vi "Remove Connection from State.vi"(8 "error in (no error)":errorcluster, 9 "Connection":T1, 10 "State":string, 11 "Channel Ref in":T2 format="%.0x") -> (0 "error out":errorcluster, 1 "connection found":bool, 3 "Channel Ref out":T2=18446744073709551615 format="%.0x")   [LabVIEW 2017, in "SLSC Switch Scripting.lvlib"]
uses:
  SLSC Switch Scripting.lvlib
  <vilib>/NI Veristand/Custom Device API/Custom Device Item Ref.ctl
  Connection.ctl
  NationalInstruments.VeriStand.SystemDefinitionAPI
  SLSC Scripting Constants.vi
  <vilib>/NI VeriStand/Custom Device API/Custom Device API.lvlib
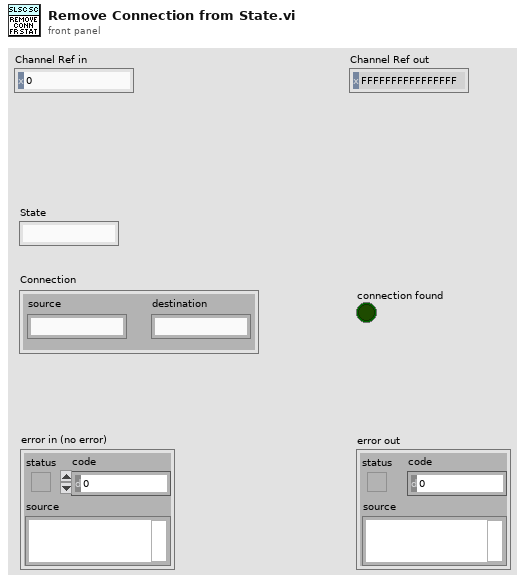
[diagram p1: front panel]
types:
  T1 = typedef "SLSC Switch Scripting.lvlib/Connection.ctl" = cluster{"source":string, "destination":string}
  T2 = typedef "Custom Device API.lvlib/Custom Device Item Ref.ctl" = u64
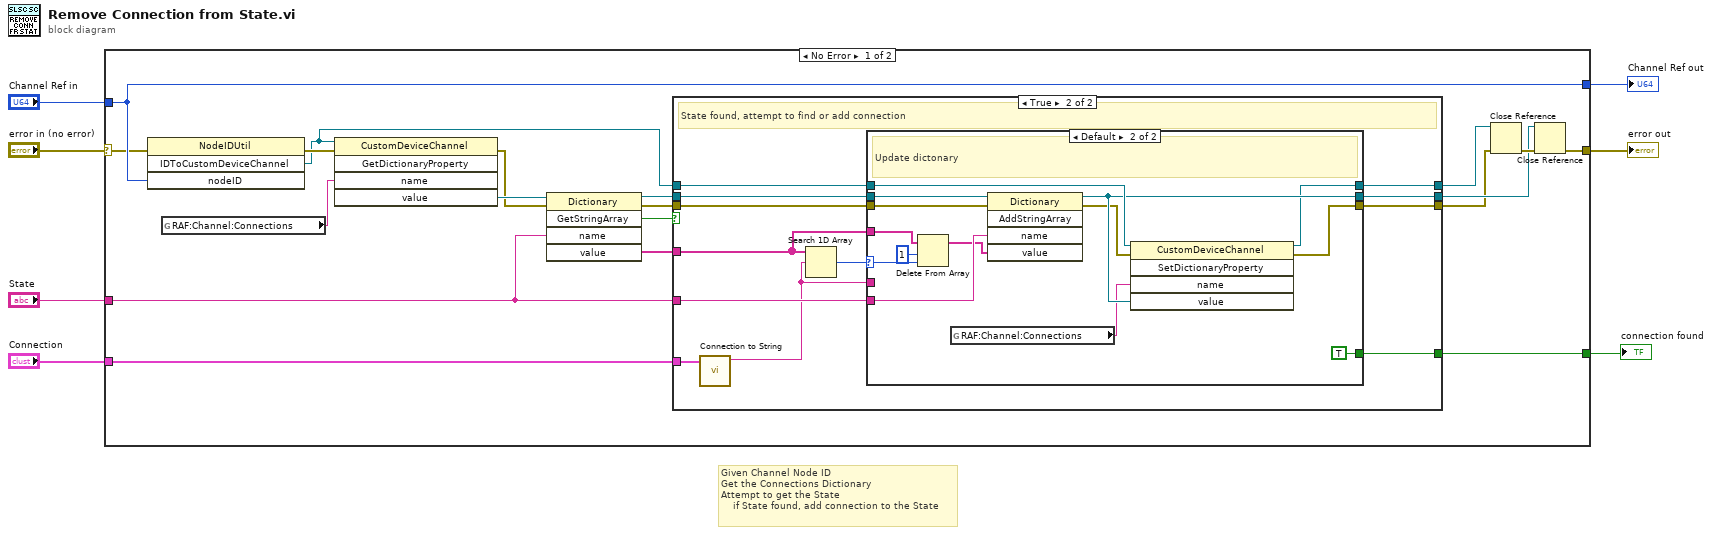
[diagram p0: block diagram]
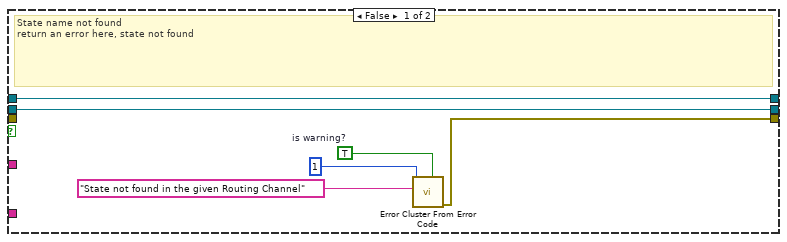
[diagram p2: hidden frame]
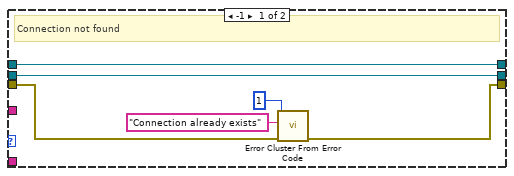
[diagram p3: hidden frame]
diagram:
  # "Given Channel Node ID\nGet the Connections Dictionary\nAttempt to get the State\n    if State found, add connection to the State"
  n1 = case shown="No Error" "error in (no error)" {
    selector: "error in (no error)" -> [w22 w66]
    tunnel: [w26 w66] -> w6
    tunnel: "Channel Ref in" -> [w23 w65]
    tunnel: [w23 w65] -> w4
    tunnel: "State" -> [w15 _]
    tunnel: [w10 _] -> w2
    tunnel: "Connection" -> [w9 _]
    frame No Error {
      n2 = invoke class="NodeIDUtil" method="IDToCustomDeviceChannel"(error in=w22, "nodeID"=w23) -> (error out=w24:errorcluster, "IDToCustomDeviceChannel"=w12:refnum<k24>)  [unwired: 2 in, 2 out]
      n3 = global read "SLSC Scripting Constants.vi" "RAF:Channel:Connections"() -> (w8:string)
      n4 = invoke class="CustomDeviceChannel" method="GetDictionaryProperty"(reference=w12, error in=w24, "name"=w8) -> (error out=w19:errorcluster, "value"=w20:refnum<k24>)  [unwired: 2 in, 3 out]
      n5 = invoke class="Dictionary" method="GetStringArray"(reference=w20, error in=w19, "name"=w15) -> (reference out=w16:refnum<k24>, error out=w17:errorcluster, "GetStringArray"=w18:bool, "value"=w21:string[])  [unwired: 2 in, 1 out]
      n6 = case shown="True" w18 {
        tunnel: w21 -> [_ w36]
        tunnel: w17 -> [_ w43]
        tunnel: [w29 w42] -> w13
        tunnel: w15 -> [_ w41]
        tunnel: w16 -> [w28 w40]
        tunnel: [w28 w39] -> w14
        tunnel: w12 -> [w27 w38]
        tunnel: [w27 w37] -> w11
        tunnel: [_ w35] -> w10
        tunnel: w9 -> [_ w34]
        frame False {
          w31 = TRUE  # is warning?
          # "State name not found\nreturn an error here, state not found"
          n7 = call <vilib>:"Error Cluster From Error Code.vi"("is warning? (False)"=w31, "error message (\"\")"="State not found in the given Routing Channel" ("error message (\"\")"), "error code (0)"=1) -> ("error out"=w29:errorcluster)  [unwired: 6 in]
        }
        frame True {
          # "State found, attempt to find or add connection"
          n8 = call "Connection to String.vi"("Connection"=w34) -> ("String"=w33:string)  [unwired: 10 in]
          n9 = Search 1D Array(1D array=w36, element=w33) -> (index of element=w44:i32)  [unwired: 1 in]
          n10 = case shown="Default" w44 {
            selector: w44 -> [_ w56]
            tunnel: w43 -> [w48 w55]
            tunnel: [w47 w59] -> w42
            tunnel: w41 -> [_ w64]
            tunnel: w40 -> [w46 w63]
            tunnel: [w46 w61] -> w39
            tunnel: w38 -> [w45 w62]
            tunnel: [w45 w58] -> w37
            tunnel: w36 -> [_ w57]
            tunnel: w33 -> [_ _]
            tunnel: [_ TRUE] -> w35
            frame -1 {
              # "Connection not found"
              n11 = call <vilib>:"Error Cluster From Error Code.vi"("error in (no error)"=w48, "error message (\"\")"="Connection already exists" ("error message (\"\")"), "error code (0)"=1) -> ("error out"=w47:errorcluster)  [unwired: 6 in]
            }
            frame Default {
              # "Update dictonary"
              n12 = Delete From Array(array=w57, length=1, index=w56) -> (array with subset deleted=w54:string[])  [unwired: 1 out]
              n13 = global read "SLSC Scripting Constants.vi" "RAF:Channel:Connections"() -> (w51:string)
              n14 = invoke class="Dictionary" method="AddStringArray"(reference=w63, error in=w55, "name"=w64, "value"=w54) -> (reference out=w61:refnum<k24>, error out=w60:errorcluster)  [unwired: 1 in, 3 out]
              n15 = invoke class="CustomDeviceChannel" method="SetDictionaryProperty"(reference=w62, error in=w60, "name"=w51, "value"=w61) -> (reference out=w58:refnum<k24>, error out=w59:errorcluster)  [unwired: 1 in, 3 out]
            }
          }
        }
      }
      n16 = Close Reference(reference=w11, error in (no error)=w13) -> (error out=w25:errorcluster)
      n17 = Close Reference(reference=w14, error in (no error)=w25) -> (error out=w26:errorcluster)
    }
    frame Error {
    }
  }
  "Channel Ref out" <- w4
  "error out" <- w6
  "connection found" <- w2
